vi "images.vi"(0 "Camera in":refnum<class "Camera.lvclass">, 1 "start_index":u32, 5 "data_format":T2(ring)=enum."Mono16", 7 "image_count":u32, 9 "roi":cluster{"x0":u64, "y0":u64, "x1":u64, "y1":u64}={"x0"=18446744073709551615, "y0"=18446744073709551615, "x1"=18446744073709551615, "y1"=18446744073709551615}, 11 "error in (no error)":errorcluster, 12 "PCO_Recorder_CompressionParams":T4={"dGainK"=nan, "dDarkNoise_e"=nan, "dDSNU_e"=nan, "dPRNU_pct"=nan, "dLightSourceNoise_pct"=0.0}) -> (2 "timestamp_list":T3(array[cluster]) {"lvTimestamp" format="%<%.6X\n%x>T"}, 3 "meta_data_list":T5(array[cluster]), 4 "Camera out":refnum<class "Camera.lvclass">, 6 "image_list (U8)":u8[][][](array[numeric]), 8 "image_list (U32)":u32[][][](array[numeric]), 10 "image_list (U64)":T1(array[cluster]), 14 "raw_image_list (U16)":u16[][][](array[numeric]), 15 "error out":errorcluster)   [LabVIEW 2019, in "Camera.lvclass"]
doc: "Get all recorded images from the recorder as a 3D array. This array is shaped depending on the\nresolution and ROI of the image and the number of recorded images. The data is stored in the\norder of image, row, column."
uses:
  Camera.lvclass
  pco.recorder/Recorder.lvlib
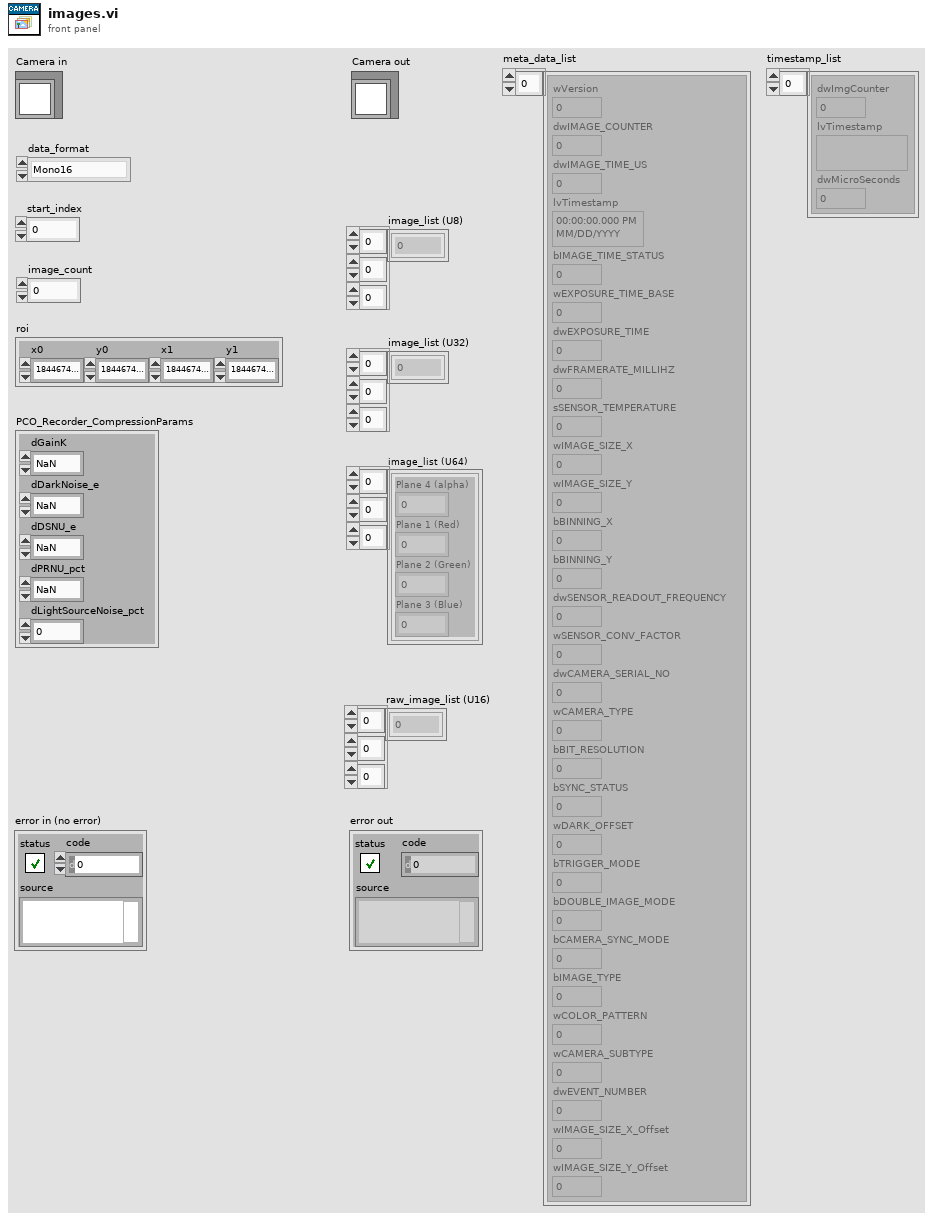
[diagram p1: front panel]
types:
  T1 = cluster{"Plane 4 (alpha)":u16, "Plane 1 (Red)":u16, "Plane 2 (Green)":u16, "Plane 3 (Blue)":u16}[][][]
  T2 = enum16{"Undefined", "Mono8", "Mono16", "BGRA8", "RGBA8", "BGRA16", "RGBA16", "CompressedMono8"}
  T3 = cluster{"dwImgCounter":u32, "lvTimestamp":timestamp, "dwMicroSeconds":u32}[]
  T4 = cluster{"dGainK":dbl, "dDarkNoise_e":dbl, "dDSNU_e":dbl, "dPRNU_pct":dbl, "dLightSourceNoise_pct":dbl}
  T5 = cluster{"wVersion":u16, "dwIMAGE_COUNTER":u32, "dwIMAGE_TIME_US":u32, "lvTimestamp":timestamp, "bIMAGE_TIME_STATUS":u8, "wEXPOSURE_TIME_BASE":u16, "dwEXPOSURE_TIME":u32, "dwFRAMERATE_MILLIHZ":u32, "sSENSOR_TEMPERATURE":i16, "wIMAGE_SIZE_X":u16, "wIMAGE_SIZE_Y":u16, "bBINNING_X":u8, "bBINNING_Y":u8, "dwSENSOR_READOUT_FREQUENCY":u32, "wSENSOR_CONV_FACTOR":u16, "dwCAMERA_SERIAL_NO":u32, "wCAMERA_TYPE":u16, "bBIT_RESOLUTION":u8, "bSYNC_STATUS":u8, "wDARK_OFFSET":u16, "bTRIGGER_MODE":u8, "bDOUBLE_IMAGE_MODE":u8, "bCAMERA_SYNC_MODE":u8, "bIMAGE_TYPE":u8, "wCOLOR_PATTERN":u16, "wCAMERA_SUBTYPE":u16, "dwEVENT_NUMBER":u32, "wIMAGE_SIZE_X_Offset":u16, "wIMAGE_SIZE_Y_Offset":u16}[]
  T6 = cluster{"dwImgCounter":u32, "lvTimestamp":timestamp, "dwMicroSeconds":u32}
  T7 = cluster{"wVersion":u16, "dwIMAGE_COUNTER":u32, "dwIMAGE_TIME_US":u32, "lvTimestamp":timestamp, "bIMAGE_TIME_STATUS":u8, "wEXPOSURE_TIME_BASE":u16, "dwEXPOSURE_TIME":u32, "dwFRAMERATE_MILLIHZ":u32, "sSENSOR_TEMPERATURE":i16, "wIMAGE_SIZE_X":u16, "wIMAGE_SIZE_Y":u16, "bBINNING_X":u8, "bBINNING_Y":u8, "dwSENSOR_READOUT_FREQUENCY":u32, "wSENSOR_CONV_FACTOR":u16, "dwCAMERA_SERIAL_NO":u32, "wCAMERA_TYPE":u16, "bBIT_RESOLUTION":u8, "bSYNC_STATUS":u8, "wDARK_OFFSET":u16, "bTRIGGER_MODE":u8, "bDOUBLE_IMAGE_MODE":u8, "bCAMERA_SYNC_MODE":u8, "bIMAGE_TYPE":u8, "wCOLOR_PATTERN":u16, "wCAMERA_SUBTYPE":u16, "dwEVENT_NUMBER":u32, "wIMAGE_SIZE_X_Offset":u16, "wIMAGE_SIZE_Y_Offset":u16}
  T8 = cluster{"Plane 4 (alpha)":u16, "Plane 1 (Red)":u16, "Plane 2 (Green)":u16, "Plane 3 (Blue)":u16}[][]
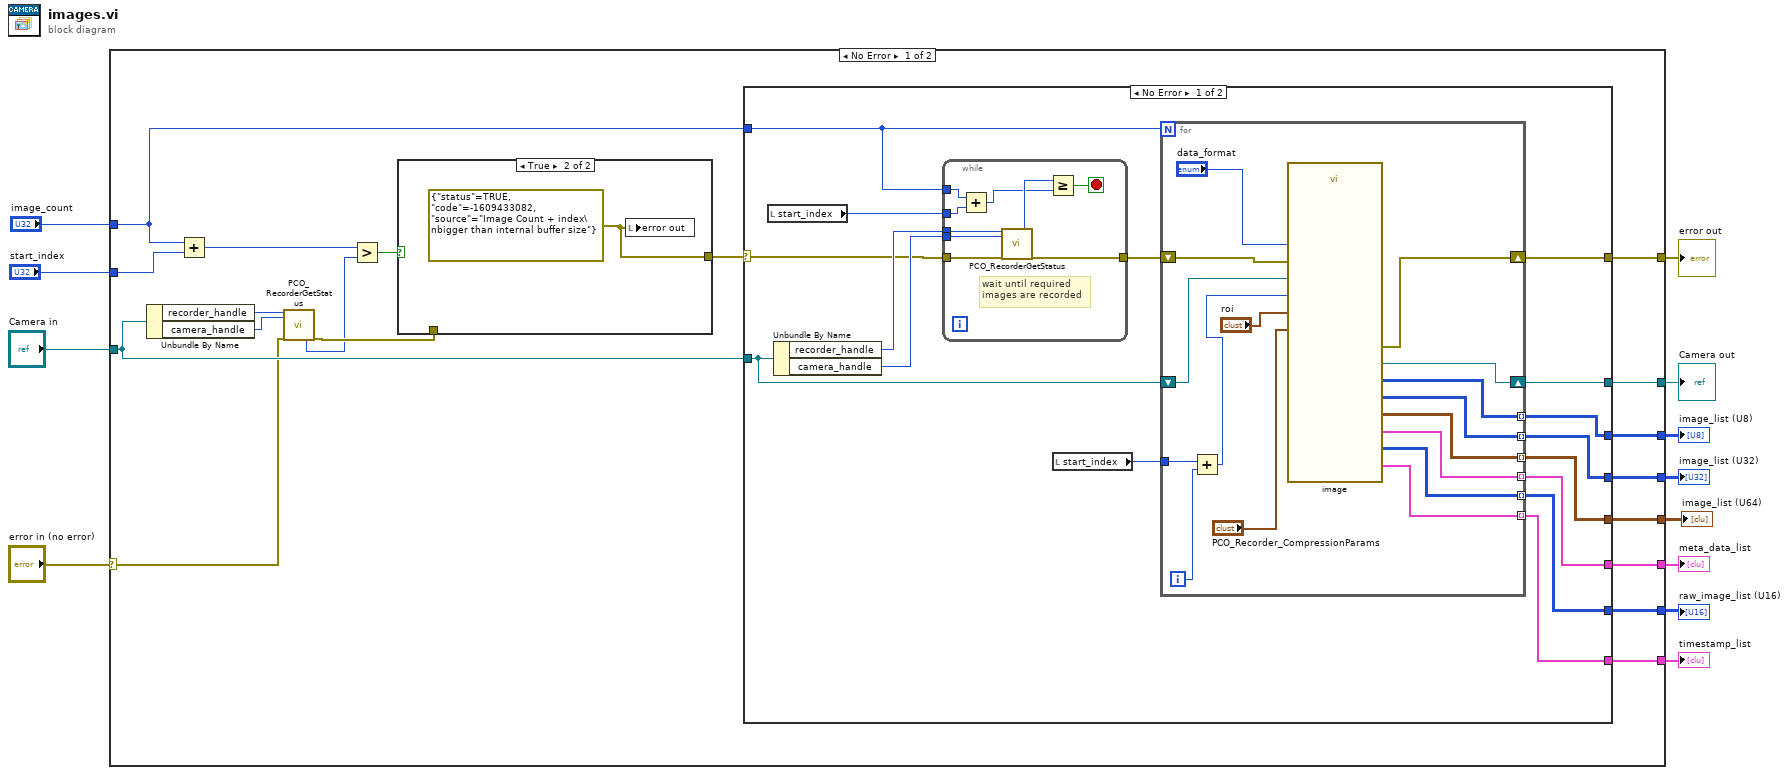
[diagram p0: block diagram]
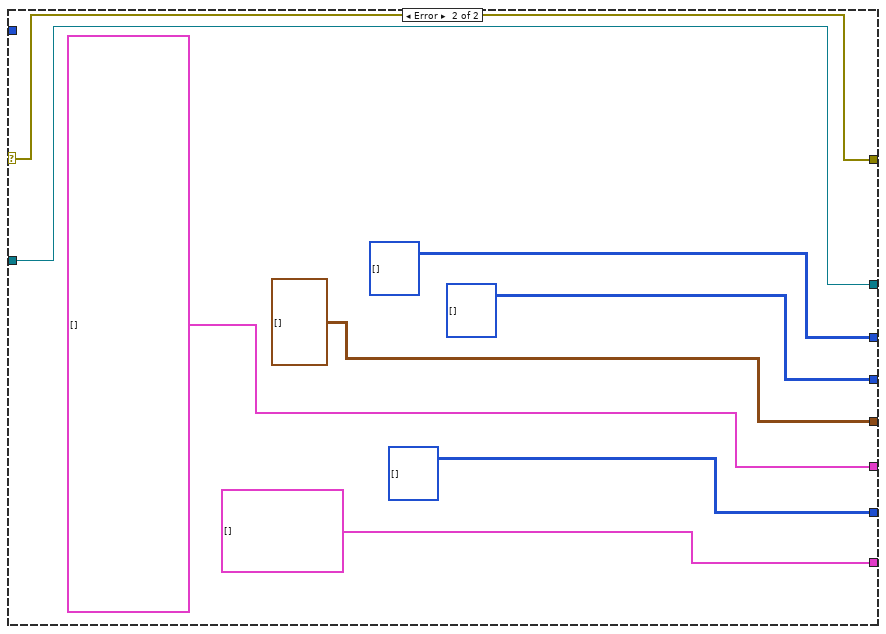
[diagram p2: hidden frame]
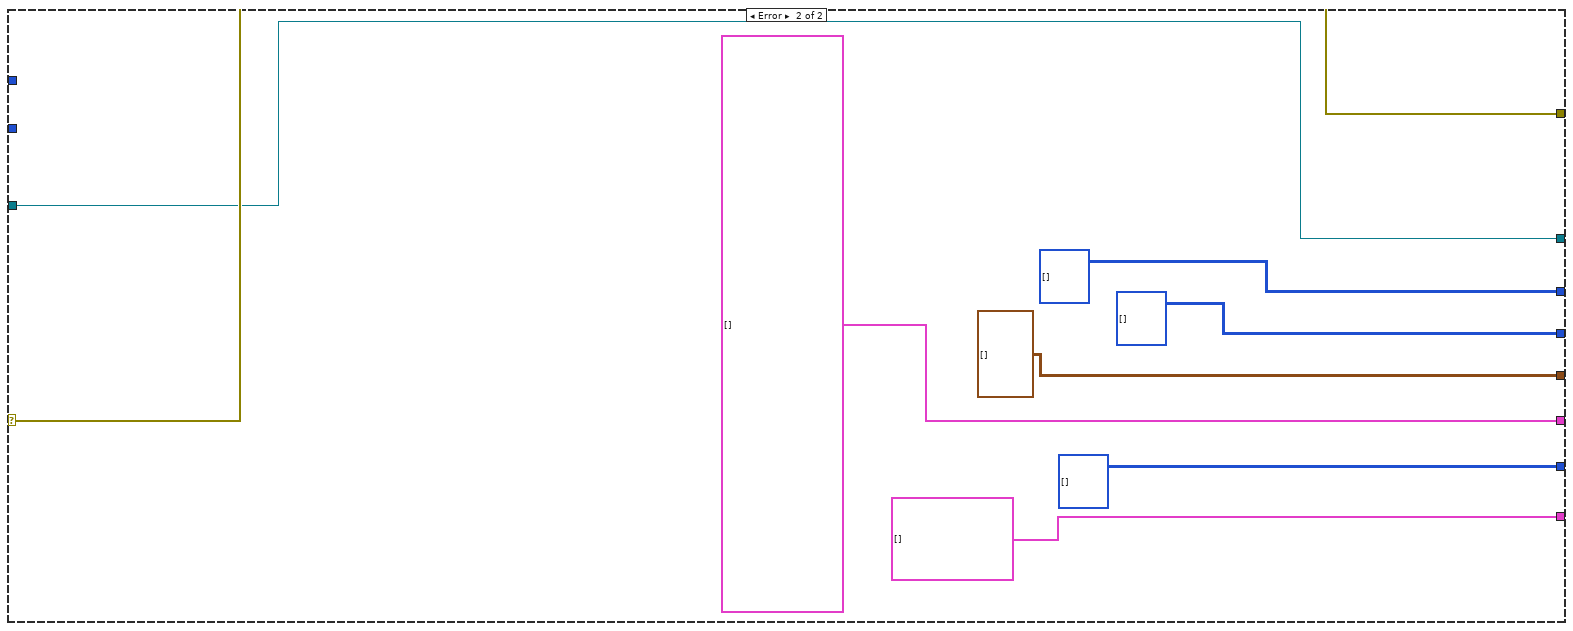
[diagram p4: hidden frame]
diagram:
  n1 = case shown="No Error" "error in (no error)" {
    selector: "error in (no error)" -> [w22 w87]
    tunnel: "Camera in" -> [w30 w86]
    tunnel: "image_count" -> [w14 _]
    tunnel: [w29 w87] -> w9
    tunnel: [w28 w86] -> w8
    tunnel: [w27 u8[][][] [] ("image (U8)")] -> w7
    tunnel: [w26 u32[][][] [] ("image (U16)")] -> w6
    tunnel: [w25 T5 []] -> w5
    tunnel: [w24 u16[][][] [] ("raw_image (U16)")] -> w4
    tunnel: [w23 T3 []] -> w3
    tunnel: "start_index" -> [w16 _]
    tunnel: [w13 T1 [] ("image (U64)")] -> w1
    frame No Error {
      n2 = Unbundle By Name(w30) -> ("recorder_handle"=w20:u64, "camera_handle"=w19:u64)
      n3 = Add(x=w14, y=w16) -> (x+y=w15:u32)
      n4 = call "PCO_RecorderGetStatus.vi"("phRec"=w20, "phCam"=w19, "error in (no error)"=w22) -> ("dwReqImgCount"=w18:u32, "error out"=w21:errorcluster)  [unwired: 5 in, 10 out]
      n5 = Greater?(x=w15, y=w18) -> (0:w31:bool)
      n6 = case shown="True" w31 {
        tunnel: [w81 w82] -> w17
        tunnel: w21 -> [w81 _]
        frame False {
        }
        frame True {
          w82 = errorcluster {"status"=TRUE, "code"=-1609433082, "source"="Image Count + index\nbigger than internal buffer size"} ("error constant")
          n7 = local write "error out"(w82) -> ()
        }
      }
      n8 = case shown="No Error" w17 {
        selector: w17 -> [w35 w80]
        tunnel: w14 -> [w45 _]
        tunnel: w30 -> [w44 w79]
        tunnel: [w42 w80] -> w29
        tunnel: [w41 w79] -> w28
        tunnel: [w36 u8[][][] [] ("image (U8)")] -> w27
        tunnel: [w40 u32[][][] [] ("image (U16)")] -> w26
        tunnel: [w32 T1 [] ("image (U64)")] -> w13
        tunnel: [w39 T5 []] -> w25
        tunnel: [w38 u16[][][] [] ("raw_image (U16)")] -> w24
        tunnel: [w37 T3 []] -> w23
        frame No Error {
          n9 = local read "start_index"() -> (w34:u32)
          n10 = Unbundle By Name(w44) -> ("recorder_handle"=w47:u64, "camera_handle"=w46:u64)
          n11 = while {
            tunnel: w47 -> [w72]
            tunnel: w46 -> [w71]
            tunnel: w35 -> [w70]
            tunnel: w45 -> [w66]
            tunnel: [w68] -> w43
            tunnel: w34 -> [w65]
            stop <- w69 stop-if-true
            # "wait until required \nimages are recorded"
            n12 = Add(x=w66, y=w65) -> (x+y=w64:u32)
            n13 = call "PCO_RecorderGetStatus.vi"("phRec"=w72, "phCam"=w71, "error in (no error)"=w70) -> ("dwProcImgCount"=w67:u32, "error out"=w68:errorcluster)  [unwired: 5 in, 10 out]
            n14 = Greater Or Equal?(x=w67, y=w64) -> (x >= y?=w69:bool)
          }
          n15 = local read "start_index"() -> (w33:u32)
          n16 = for {
            N: w45 -> [_]
            shift-right: [w60] -> w42
            shift-left: w43 -> [w61]
            shift-right: [w59] -> w41
            shift-left: w44 -> [w63]
            tunnel: [w58] -> w40 mode=indexing
            tunnel: [w57] -> w36 mode=indexing
            tunnel: [w56] -> w32 mode=indexing
            tunnel: [w55] -> w39 mode=indexing
            tunnel: [w54] -> w38 mode=indexing
            tunnel: [w51] -> w37 mode=indexing
            tunnel: w33 -> [w49]
            i -> [w50]
            n17 = Add(x=w49, y=w50) -> (x+y=w48:u32)
            n18 = call-dynamic "image.vi"("Camera in"=w63, "data_format"="data_format", "image_index"=w48, "roi"="roi", "error in (no error)"=w61, "PCO_Recorder_CompressionParams"="PCO_Recorder_CompressionParams") -> ("timestamp"=w51:T6, "meta_data"=w55:T7, "Camera out"=w59:refnum<class "Camera.lvclass">, "image (U8)"=w57:u8[][], "image (U32)"=w58:u32[][], "image (U64)"=w56:T8, "raw_image (U16)"=w54:u16[][], "error out"=w60:errorcluster)  [unwired: 2 in]
          }
        }
        frame Error {
        }
      }
    }
    frame Error {
    }
  }
  "error out" <- w9
  "Camera out" <- w8
  "meta_data_list" <- w5
  "timestamp_list" <- w3
  "raw_image_list (U16)" <- w4
  "image_list (U32)" <- w6
  "image_list (U8)" <- w7
  "image_list (U64)" <- w1
